vi "Check array equality.vi"(8 "error in (no error)":errorcluster, 9 "Equal and clusters?":bool, 10 "Element to be inserted":variant, 11 "Upper Level Cluster Ele":variant) -> (0 "error out":errorcluster, 3 "Equal?":bool)   [LabVIEW 2015]
uses:
  <vilib>/Utility/Data Type/NI_Data Type.lvlib
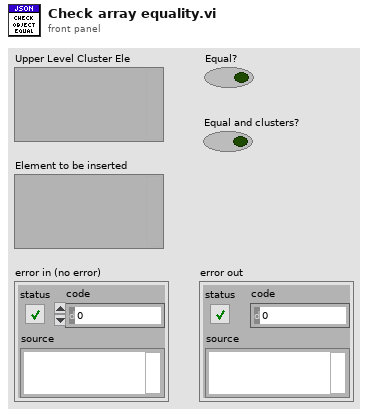
[diagram p1: front panel]
types:
  T1 = typedef "NI_Data Type.lvlib/Data Type.ctl" = enum8{"Invalid Type", "Void", "I8", "I16", "I32", "I64", "U8", "U16", "U32", "U64", "Single Float", "Double Float", "Extended Float", "Single Complex", "Double Complex", "Extended Complex", "Enum U8", "Enum U16", "Enum U32", "Enum U64", "Single Float With Unit", "Double Float With Unit", "Extended Float With Unit", "Single Complex with Unit", "Double Complex with Unit", "Extended Complex with Unit", "Boolean", "String", "Path", "Picture", "Tag", "Array", "Cluster", "Variant", "LV Variant", "Waveform", "Timestamp", "Digital Waveform", "Digital Data", "ExpressData", "Refnum", "External Data", "VI", "Poly VI", "LabVIEW Class Instance", "Fixed Point"}
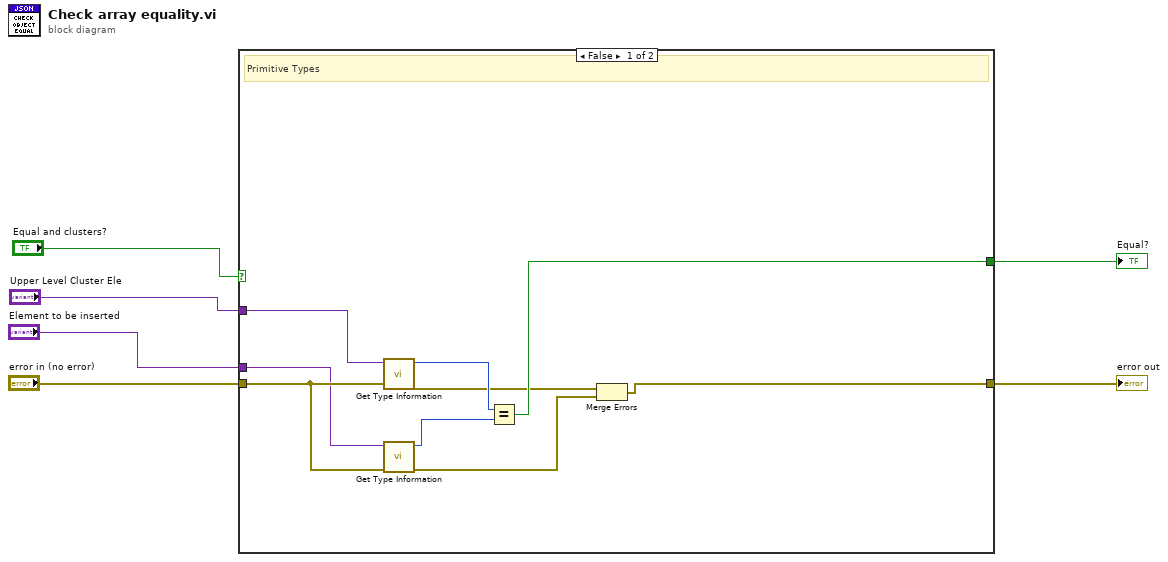
[diagram p0: block diagram]
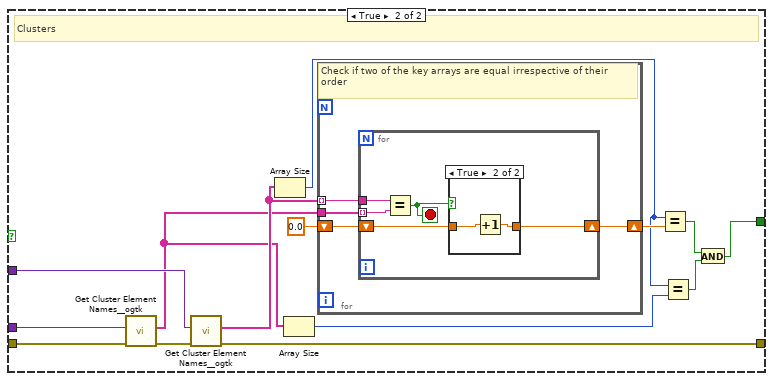
[diagram p2: hidden frame]
diagram:
  n1 = case shown="False" "Equal and clusters?" {
    tunnel: "Upper Level Cluster Ele" -> [w14 w29]
    tunnel: [w10 w16] -> w5
    tunnel: [w7 w24] -> w4
    tunnel: "Element to be inserted" -> [w13 w23]
    tunnel: "error in (no error)" -> [w15 w22]
    frame False {
      # "Primitive Types"
      n2 = call <vilib>:"Get Type Information.vi"("error in (no error)"=w15, "Variant"=w14) -> ("error out"=w9:errorcluster, "Type"=w11:T1)  [unwired: 5 in, 3 out]
      n3 = call <vilib>:"Get Type Information.vi"("error in (no error)"=w15, "Variant"=w13) -> ("error out"=w8:errorcluster, "Type"=w12:T1)  [unwired: 5 in, 3 out]
      n4 = Equal?(x=w11, y=w12) -> (x = y?=w10:bool)
      n5 = Merge Errors(w9, w8) -> (w7:errorcluster)
    }
    frame True {
      # "Clusters"
      n6 = call <userlib>:"Get Cluster Element Names__ogtk.vi"("error in (no error)"=w22, "Cluster"=w23) -> ("error out"=w25:errorcluster, "Element Names"=w21:string[])  [unwired: 8 in]
      n7 = call <userlib>:"Get Cluster Element Names__ogtk.vi"("error in (no error)"=w25, "Cluster"=w29) -> ("error out"=w24:errorcluster, "Element Names"=w27:string[])  [unwired: 8 in]
      n8 = Array Size(array=w27) -> (size(s)=w20:i32)
      n9 = Array Size(array=w21) -> (size(s)=w19:i32)
      n10 = for {
        tunnel: w27 -> [w33] mode=indexing
        tunnel: w21 -> [w32]
        shift-right: [w31] -> w28
        shift-left: 0.0 -> [w30]
        # "Check if two of the key arrays are equal irrespective of their order"
        n11 = for {
          tunnel: w33 -> [w38]
          tunnel: w32 -> [w37] mode=indexing
          shift-right: [w36] -> w31
          shift-left: w30 -> [w35]
          stop <- w34 stop-if-true
          n12 = Equal?(x=w38, y=w37) -> (x = y?=w34:bool)
          n13 = case shown="True" w34 {
            tunnel: [w39 w41] -> w36
            tunnel: w35 -> [w39 w40]
            frame False {
            }
            frame True {
              n14 = Increment(x=w40) -> (x+1=w41:dbl)
            }
          }
        }
      }
      n15 = Equal?(x=w20, y=w28) -> (x = y?=w17:bool)
      n16 = Equal?(x=w20, y=w19) -> (x = y?=w18:bool)
      n17 = And(x=w17, y=w18) -> (x .and. y?=w16:bool)
    }
  }
  "Equal?" <- w5
  "error out" <- w4
